vi "Persist Element.vi"(8 "error in (no error)":errorcluster, 9 "Parent":i32, 10 "Element":refnum<class "Config Element.lvclass">, 11 "Config-Sqlite in":refnum<class "Config-Sqlite.lvclass">) -> (0 "error out":errorcluster, 2 "Row":i32, 3 "Config-Sqlite out":refnum<class "Config-Sqlite.lvclass">)   [LabVIEW 2020, in "CDM-Config.lvlib" / "Config-Sqlite.lvclass"]
uses:
  Config-Sqlite.lvclass
  C:/dev/lv20CE/lv-cdm/CDM-Config/Config Storage/Config Storage.lvclass
  Config Element/Config Element.lvclass
  Config-Sqlite.lvclass/Config-Sqlite.ctl
  <vilib>/drjdpowell/SQLite Library/SQL Statement/SQL Statement.lvclass/SQL Statement.ctl
  <vilib>/drjdpowell/SQLite Library/SQL Connection/Connection.lvclass/Connection.ctl
  <vilib>/drjdpowell/SQLite Library/SQL Statement/Bind Text.vi
  <vilib>/drjdpowell/SQLite Library/SQL Statement/Bind Integer.vi
  <vilib>/drjdpowell/SQLite Library/SQL Statement/Step.vi
  <vilib>/drjdpowell/SQLite Library/SQL Statement/Error Message.vi
  <vilib>/drjdpowell/SQLite Library/SQL Connection/Connection.lvclass
  <vilib>/drjdpowell/SQLite Library/SQL Statement/SQL Statement.lvclass
  Config Storage/Config Storage.lvclass
panel:
  out "Row 2":i32
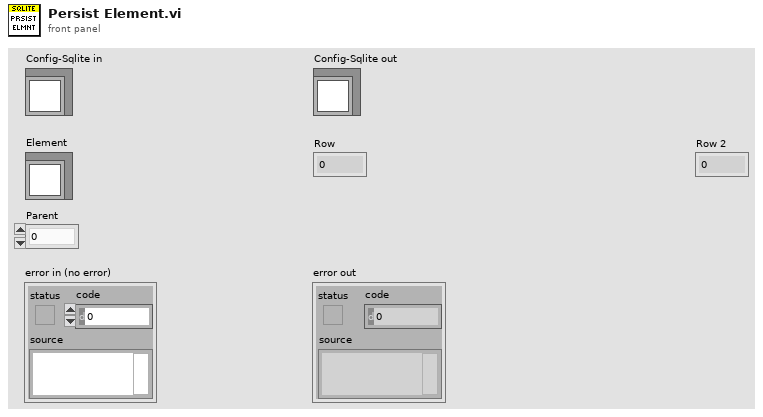
[diagram p1: front panel]
types:
  T1 = typedef "CDM-Config.lvlib/Meta Data.ctl" = cluster{"Name":string, "Value":string}
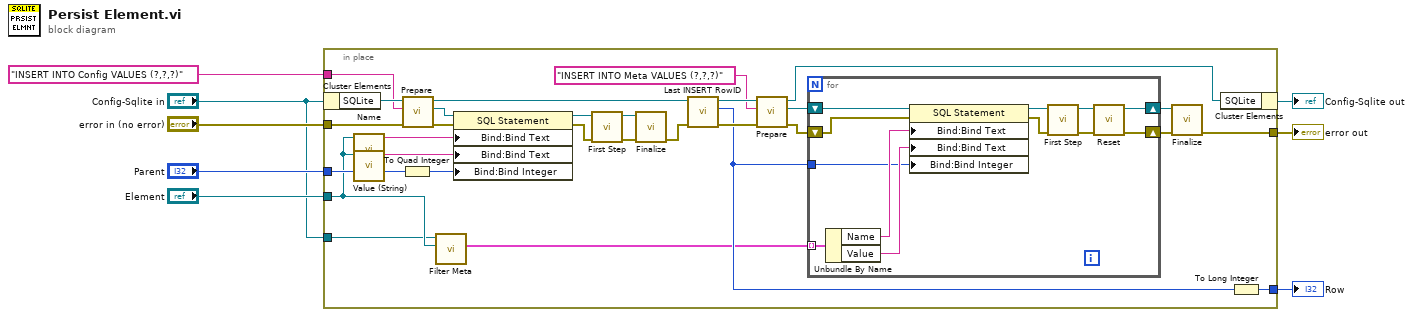
[diagram p0: block diagram]
diagram:
  n1 = in-place {
    in-place-border: "Element" -> [w10]
    in-place-border: "Parent" -> [w31]
    in-place-border: "INSERT INTO Config VALUES (?,?,?)" -> [w36]
    in-place-border: [w21] -> w4
    in-place-border: "error in (no error)" -> [w14]
    in-place-border: [w13] -> w2
    in-place-border: "Config-Sqlite in" -> [w9]
    n2 = in-place-cluster #1("Config-Sqlite in") -> ("SQLite"=w37:refnum<class "Connection.lvclass">)
    n3 = call "Name.vi"("Config Element in"=w10) -> ("Name"=w34:string)  [unwired: 9 in, 1 out]
    n4 = call "Value (String).vi"("Config Element in"=w10) -> ("String Value"=w32:string)  [unwired: 9 in, 1 out]
    n5 = To Quad Integer(1:w31) -> (0:w30:i64)
    n6 = call <vilib>:"Prepare.vi"("error in (no error)"=w14, "SQL"=w36, "SQLite Connection in"=w37) -> ("error out"=w33:errorcluster, "SQL Statement"=w35:refnum<class "SQL Statement.lvclass">, "SQLite Connection"=w25:refnum<class "Connection.lvclass">)  [unwired: 4 in, 2 out]
    n7 = call "Filter Meta.vi"("Element"=w10, "Config Storage in"=w9) -> ("Filtered Meta"=w11:T1[])  [unwired: 7 in, 2 out]
    n8 = property class="SQL Statement"(reference=w35, error in=w33, "Bind:Bind Text"=w34, "Bind:Bind Text"=w32, "Bind:Bind Integer"=w30) -> (reference out=w29:refnum<class "SQL Statement.lvclass">, error out=w28:errorcluster)
    n9 = call <vilib>:"First Step.vi"("error in (no error)"=w28, "SQL Statement in"=w29) -> ("error out"=w27:errorcluster, "SQL Statement"=w26:refnum<class "SQL Statement.lvclass">)  [unwired: 7 in, 1 out]
    n10 = call <vilib>:"Finalize.vi"("error in (no error)"=w27, "SQL Statement in"=w26) -> ("error out"=w24:errorcluster)  [unwired: 9 in]
    n11 = call <vilib>:"Last INSERT RowID.vi"("error in (no error)"=w24, "SQLite Connection in"=w25) -> ("error out"=w22:errorcluster, "Last INSERT RowID"=w20:i64, "SQLite Connection"=w23:refnum<class "Connection.lvclass">)  [unwired: 7 in]
    n12 = call <vilib>:"Prepare.vi"("error in (no error)"=w22, "SQL"="INSERT INTO Meta VALUES (?,?,?)", "SQLite Connection in"=w23) -> ("error out"=w18:errorcluster, "SQL Statement"=w17:refnum<class "SQL Statement.lvclass">, "SQLite Connection"=w12:refnum<class "Connection.lvclass">)  [unwired: 4 in, 2 out]
    n13 = for {
      tunnel: w20 -> [w44]
      shift-right: [w38] -> w15
      shift-left: w18 -> [w48]
      shift-right: [w39] -> w16
      shift-left: w17 -> [w49]
      tunnel: w11 -> [w47] mode=indexing
      n14 = Unbundle By Name(w47) -> ("Name"=w46:string, "Value"=w45:string)
      n15 = property class="SQL Statement"(reference=w49, error in=w48, "Bind:Bind Text"=w46, "Bind:Bind Text"=w45, "Bind:Bind Integer"=w44) -> (reference out=w43:refnum<class "SQL Statement.lvclass">, error out=w42:errorcluster)
      n16 = call <vilib>:"First Step.vi"("error in (no error)"=w42, "SQL Statement in"=w43) -> ("error out"=w41:errorcluster, "SQL Statement"=w40:refnum<class "SQL Statement.lvclass">)  [unwired: 7 in, 1 out]
      n17 = call <vilib>:"Reset.vi"("error in (no error)"=w41, "SQL Statement in"=w40) -> ("error out"=w38:errorcluster, "SQL Statement"=w39:refnum<class "SQL Statement.lvclass">)  [unwired: 8 in]
    }
    n18 = call <vilib>:"Finalize.vi"("error in (no error)"=w15, "SQL Statement in"=w16) -> ("error out"=w13:errorcluster)  [unwired: 9 in]
    n19 = in-place-cluster #1("SQLite"=w12) -> (→"Config-Sqlite out":refnum<class "Config-Sqlite.lvclass">)
    n20 = To Long Integer(number=w20) -> (32bit integer=w21:i32)
  }
  "error out" <- w2
  "Row" <- w4
